vi "Hormiga_ReadPort.vi"(8 "error in (no error)":errorcluster, 10 "Puerto":enum32{"PORTB", "PORTD"}(ring), 11 "VISA Refnum in":refnum<visa-resource-name>) -> (0 "error out":errorcluster, 2 "Value":u16, 3 "VISA Refnum out":refnum<visa-resource-name>)   [LabVIEW 2016]
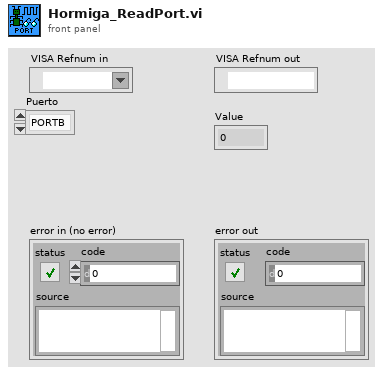
[diagram p1: front panel]
types:
  T1 = enum16{"pinMode", "digitalWrite", "digitalRead", "analogRead", "analogWrite", "PBRead", "ReadPort", "WritePort", "ReadUS", "TrisPORT"}
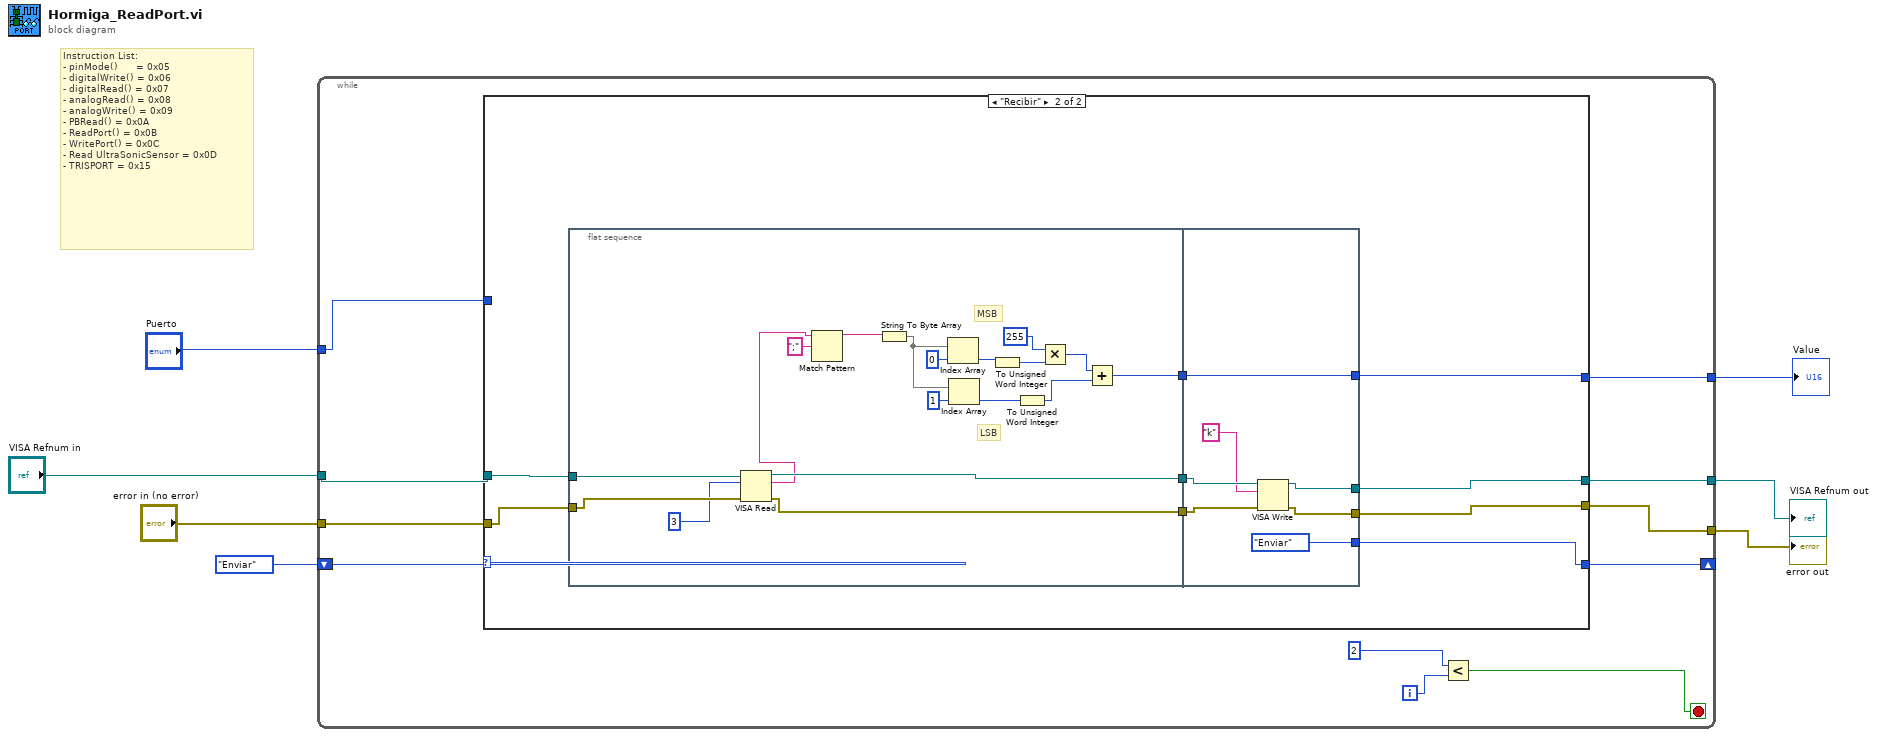
[diagram p0: block diagram]
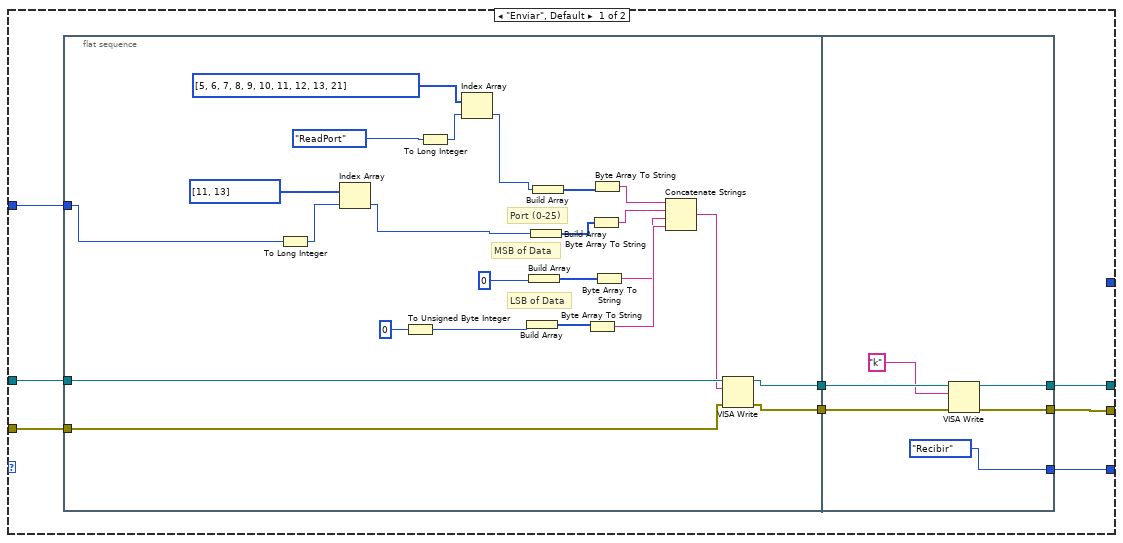
[diagram p2: hidden frame]
diagram:
  # "Instruction List:\n- pinMode()      = 0x05\n- digitalWrite() = 0x06\n- digitalRead() = 0x07\n- analogRead() = 0x08\n- analogWrite() = 0x09 \n- PBRead() = 0x0A\n- ReadPort() = 0x0B\n- WritePort() = 0x0C\n- Read UltraSonicSensor = 0x0D\n- TRISPORT = 0x15"
  n1 = while {
    shift-right: [w13] -> _
    shift-left: enum16{"Enviar", "Recibir"}."Enviar" -> [w18]
    tunnel: "error in (no error)" -> [w17]
    tunnel: "VISA Refnum in" -> [w16]
    tunnel: [w15] -> w4
    tunnel: [w14] -> w5
    tunnel: "Puerto" -> [w9]
    tunnel: [w8] -> w7
    i -> [w11]
    stop <- w12 stop-if-true
    n2 = case shown="\"Recibir\"" w18 {
      tunnel: w17 -> [w26 w65]
      tunnel: w16 -> [w25 w64]
      tunnel: [w22 w61] -> w15
      tunnel: [w21 w60] -> w14
      tunnel: [w20 w59] -> w13
      tunnel: w9 -> [w19 _]
      tunnel: [_ w57] -> w8
      frame "Enviar", Default {
        n3 = flat-sequence {
          tunnel: w26 -> [w50]
          tunnel: w25 -> [w49]
          tunnel: [w48] -> w24
          tunnel: [w47] -> w23
          tunnel: w19 -> [w31]
          tunnel: w24 -> [w56]
          tunnel: w23 -> [w55]
          tunnel: [w53] -> w22
          tunnel: [w52] -> w21
          tunnel: [enum16{"Enviar", "Recibir"}."Recibir"] -> w20
          frame #0 {
            # "LSB of Data"
            # "MSB of Data"
            # "Port (0-25)"
            n4 = To Long Integer(number=w31) -> (32bit integer=w33:i32)
            n5 = Index Array(array=u8[] [11, 13], index=w33) -> (element=w32:u8)
            n6 = To Unsigned Byte Integer(number=u8 0) -> (unsigned 8bit integer=w36:u8)
            n7 = To Long Integer(number=T1."ReadPort") -> (32bit integer=w28:i32)
            n8 = Index Array(array=u8[] [5, 6, 7, 8, 9, 10, 11, 12, 13, 21], index=w28) -> (element=w27:u8)
            n9 = Build Array(w36) -> (w42:u8[])
            n10 = Build Array(u8 0) -> (w43:u8[])
            n11 = Build Array(w32) -> (w44:u8[])
            n12 = Build Array(w27) -> (w45:u8[])
            n13 = Byte Array To String(unsigned byte array=w42) -> (string=w41:string)
            n14 = Byte Array To String(unsigned byte array=w44) -> (string=w39:string)
            n15 = Byte Array To String(unsigned byte array=w45) -> (string=w38:string)
            n16 = Byte Array To String(unsigned byte array=w43) -> (string=w40:string)
            n17 = Concatenate Strings(w38, w39, w40, w41) -> (w37:string)
            n18 = VISA Write(VISA resource name=w49, write buffer=w37, error in (no error)=w50) -> (VISA resource name out=w47:refnum<visa-resource-name>, error out=w48:errorcluster)  [unwired: 1 out]
          }
          frame #1 {
            n19 = VISA Write(VISA resource name=w55, write buffer="k", error in (no error)=w56) -> (VISA resource name out=w52:refnum<visa-resource-name>, error out=w53:errorcluster)  [unwired: 1 out]
          }
        }
      }
      frame "Recibir" {
        n20 = flat-sequence {
          tunnel: w65 -> [w75]
          tunnel: w64 -> [w74]
          tunnel: [w83] -> w63
          tunnel: [w82] -> w62
          tunnel: [w76] -> w58
          tunnel: w63 -> [w90]
          tunnel: w62 -> [w89]
          tunnel: [w87] -> w61
          tunnel: [w86] -> w60
          tunnel: [enum16{"Enviar", "Recibir"}."Enviar"] -> w59
          tunnel: w58 -> [w84]
          tunnel: [w84] -> w57
          frame #0 {
            # "MSB"
            # "LSB"
            n21 = VISA Read(VISA resource name=w74, byte count=u32 3, error in (no error)=w75) -> (VISA resource name out=w82:refnum<visa-resource-name>, read buffer=w66:string, error out=w83:errorcluster)  [unwired: 1 out]
            n22 = Match Pattern(string=w66, regular expression=";") -> (before substring=w68:string)  [unwired: 1 in, 3 out]
            n23 = String To Byte Array(string=w68) -> (unsigned byte array=w81:u8[])
            n24 = Index Array(array=w81, index=0) -> (element=w70:u8)
            n25 = Index Array(array=w81, index=1) -> (element=w72:u8)
            n26 = To Unsigned Word Integer(number=w70) -> (unsigned 16bit integer=w69:u16)
            n27 = To Unsigned Word Integer(number=w72) -> (unsigned 16bit integer=w71:u16)
            n28 = Multiply(x=u16 255, y=w69) -> (x*y=w78:u16)
            n29 = Add(x=w78, y=w71) -> (x+y=w76:u16)
          }
          frame #1 {
            n30 = VISA Write(VISA resource name=w89, write buffer="k", error in (no error)=w90) -> (VISA resource name out=w86:refnum<visa-resource-name>, error out=w87:errorcluster)  [unwired: 1 out]
          }
        }
      }
    }
    n31 = Less?(x=2, y=w11) -> (x < y?=w12:bool)
  }
  "Value" <- w7
  "VISA Refnum out" <- w5
  "error out" <- w4
